vi "Write.vi"(8 "error in":errorcluster, 10 "Variant":variant, 11 "Reply Protocol DataSocket in":refnum<class "Reply Protocol DataSocket.lvclass">) -> (0 "error out":errorcluster, 1 "timed out":bool, 3 "Reply Protocol DataSocket out":refnum<class "Reply Protocol DataSocket.lvclass">)   [LabVIEW 2023, in "HAL GOOP4.lvlib" / "Reply Protocol DataSocket.lvclass"]
uses:
  Reply Protocol DataSocket.lvclass
  Reply Protocol DataSocket.lvclass/Reply Protocol DataSocket.ctl
  Reply Protocol Base/Reply Protocol Base.lvclass
  D:/git/HAL/HAL GOOP4/Reply Protocol/Reply Protocol Base/Reply Protocol Base.lvclass
  D:/git/HAL/HAL GOOP4/Reply Protocol/Reply Protocol DataSocket/Reply Protocol DataSocket.lvclass
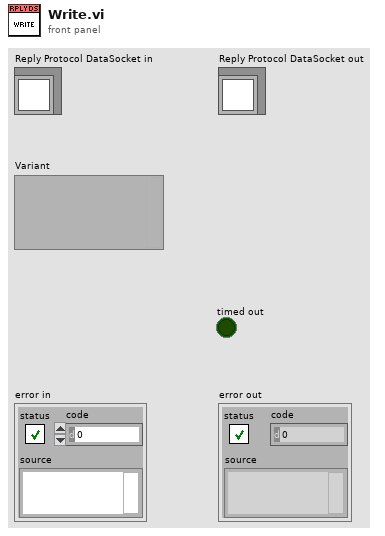
[diagram p1: front panel]
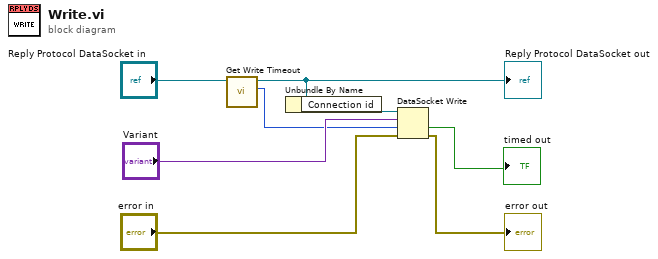
[diagram p0: block diagram]
diagram:
  n1 = call "Get Write Timeout.vi"("Reply Protocol Base in"="Reply Protocol DataSocket in") -> ("Write Timeout"=w1:i32, "Reply Protocol Base out"=w5:refnum<class "Reply Protocol DataSocket.lvclass">)  [unwired: 9 in]
  "Reply Protocol DataSocket out" <- w5
  n2 = Unbundle By Name(w5) -> ("Connection id"=w2:refnum<k13>)
  n3 = DataSocket Write(8:"error in", 9:w1, 10:"Variant", 11:w2) -> (0:→"error out":errorcluster, 1:→"timed out":bool)  [unwired: 1 out]
